vi "串口配置.vi"(8 "PORT":string="1001", 9 "IP":string="127.0.0.1", 10 "MB通信方式选择":enum16{"串口", "TCP"}(ring), 11 "请选择串口:":refnum<visa-resource-name>) -> (0 "PORT 2":string="1001", 1 "IP 2":string="127.0.0.1", 2 "确认 2":bool, 3 "VISA资源名称 2":refnum<visa-resource-name>, 4 "MB通信方式选择 2":enum16{"串口", "TCP"}(ring))   [LabVIEW 2016, in "斯坦道氟化物.lvlib"]
uses:
  <vilib>/Utility/miscctls.llb/LVPointTypeDef.ctl
panel:
  out "MB table":enum32{"Serial", "TCP"}(tab)
  in  "取消":bool
  in  "确认":bool
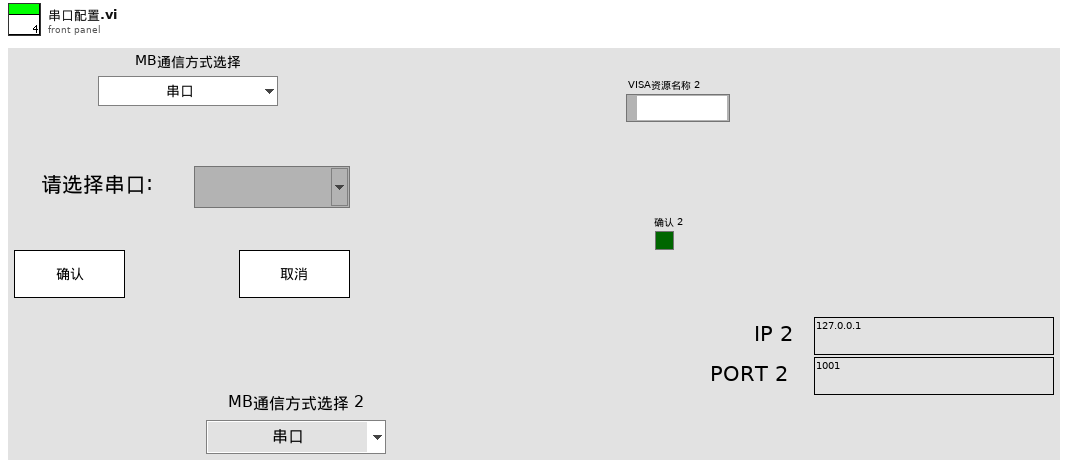
[diagram p1: front panel]
types:
  T1 = typedef "LVPointTypeDef.ctl" = cluster{"Horizontal":i16, "Vertical":i16}
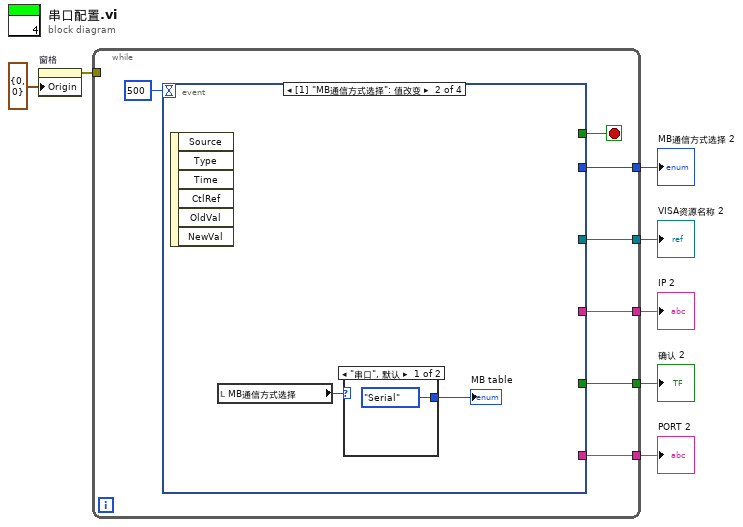
[diagram p0: block diagram]
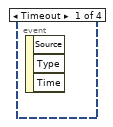
[diagram p2: hidden frame]
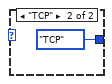
[diagram p3: hidden frame]
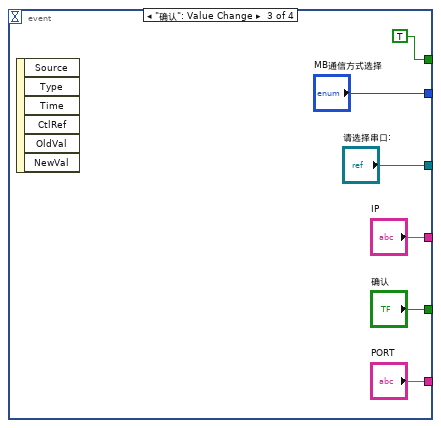
[diagram p4: hidden frame]
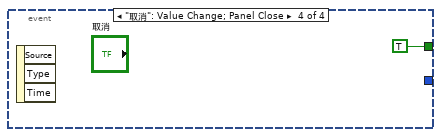
[diagram p5: hidden frame]
diagram:
  n1 = property on="窗格" class="Pane"("Origin"=T1 {"Horizontal"=0, "Vertical"=0} ("原点")) -> (error out=w1:errorcluster)  [unwired: 2 in, 1 out]
  n2 = while {
    tunnel: [w14] -> w7
    tunnel: [w12] -> w6
    tunnel: [w11] -> w5
    tunnel: [w10] -> w4
    tunnel: [w9] -> w3
    tunnel: w1 -> [_]
    stop <- w13 stop-if-true
    n3 = event shown="[1] \"MB通信方式选择\": 值改变" {
      selector: _ -> [_ _ _ _]
      dyn-events: _ -> [_ _ _ _]
      timeout: 500 -> [_ _ _ _]
      tunnel: [_ _ "请选择串口:" _] -> w14
      tunnel: [_ _ TRUE TRUE] -> w13
      tunnel: [_ _ "确认" _] -> w12
      tunnel: [_ _ "IP" _] -> w11
      tunnel: [_ _ "PORT" _] -> w10
      tunnel: [_ _ "MB通信方式选择" _] -> w9
      event Timeout {
        n4 = event-data() -> ()  [unwired: 1 in, 3 out]
      }
      event "MB通信方式选择": Value Change {
        n5 = event-data() -> ()  [unwired: 1 in, 6 out]
        n6 = local read "MB通信方式选择"() -> (w16:enum16{"串口", "TCP"})
        n7 = case shown="\"串口\", 默认" w16 {
          tunnel: [enum32{"Serial", "TCP"}."Serial" ("MB table") enum32{"Serial", "TCP"}."TCP" ("MB table")] -> w15
          frame "串口", Default {
          }
          frame "TCP" {
          }
        }
        "MB table" <- w15
      }
      event "确认": Value Change {
        n8 = event-data() -> ()  [unwired: 1 in, 6 out]
      }
      event "取消": Value Change; Panel Close {
        n9 = event-data() -> ()  [unwired: 1 in, 3 out]
      }
    }
  }
  "VISA资源名称 2" <- w7
  "确认 2" <- w6
  "IP 2" <- w5
  "PORT 2" <- w4
  "MB通信方式选择 2" <- w3
